vi "no error.vi"(3 "error in (no error)":errorcluster) -> (0 "error out":errorcluster)   [LabVIEW 2026, in "MicroPulse_Driver.lvlib"]
uses:
  MicroPulse_Driver.lvlib
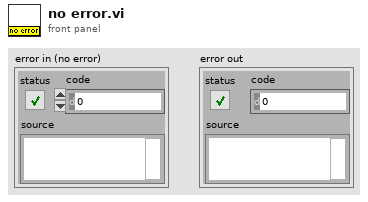
[diagram p1: front panel]
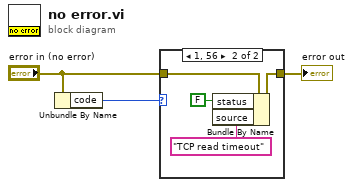
[diagram p0: block diagram]
diagram:
  n1 = Unbundle By Name("error in (no error)") -> ("code"=w1:i32)
  n2 = case shown="1, 56" w1 {
    tunnel: [w4 w8] -> w3
    tunnel: "error in (no error)" -> [w4 w7]
    frame Default {
    }
    frame 1, 56 {
      n3 = Bundle By Name(cluster=w7, "status"=FALSE, "source"="TCP read timeout") -> (w8:errorcluster)
    }
  }
  "error out" <- w3
